vi "Get Settings.vi"(10 "VI path":path, 11 "switches":cluster{"switch":string, "argument":string}[](array[cluster])) -> (3 "settings":T1)   [LabVIEW 2017]
doc: "Prepares information necessary to create a new icon."
uses:
  CTLs/Settings.ctl
  CTLs/Template Frame.ctl
  CTLs/Text Format.ctl
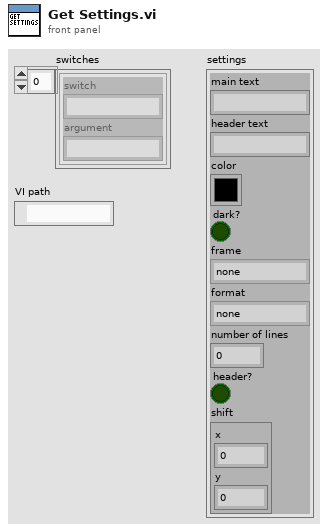
[diagram p1: front panel]
types:
  T1 = typedef "Settings.ctl" = cluster{"main text":string, "header text":string, "color":u32, "dark?":bool, "frame":T2, "format":T3, "number of lines":i32, "header?":bool, "shift":cluster{"x":i16, "y":i16}}
  T2 = typedef "Template Frame.ctl" = enum16{"none", "compact lib"}
  T3 = typedef "Text Format.ctl" = enum16{"none"}
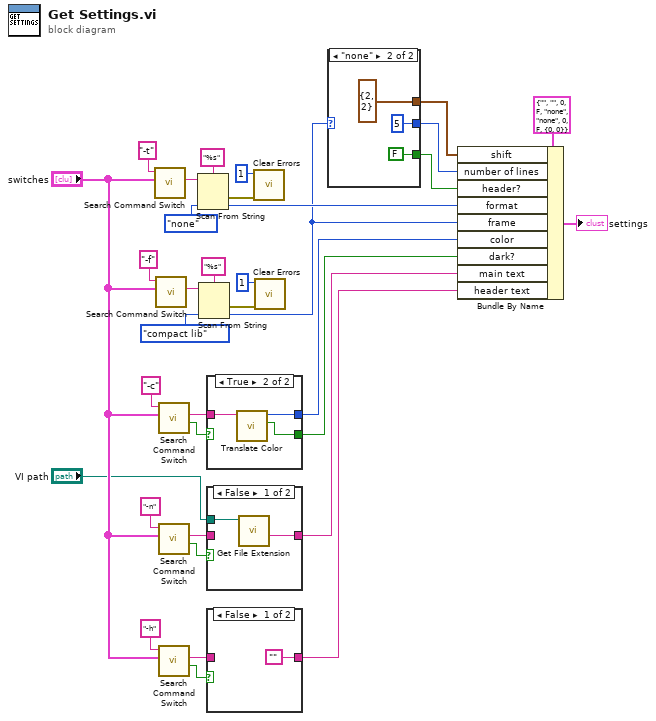
[diagram p0: block diagram]
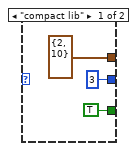
[diagram p2: hidden frame]
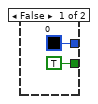
[diagram p5: hidden frame]
diagram:
  n1 = call "Search Command Switch.vi"("switches"="switches", "switch in"="-t") -> ("argument"=w22:string)  [unwired: 7 in, 2 out]
  n2 = call "Search Command Switch.vi"("switches"="switches", "switch in"="-f") -> ("argument"=w33:string)  [unwired: 7 in, 2 out]
  n3 = call "Search Command Switch.vi"("switches"="switches", "switch in"="-c") -> ("found?"=w26:bool, "argument"=w27:string)  [unwired: 7 in, 1 out]
  n4 = call "Search Command Switch.vi"("switches"="switches", "switch in"="-n") -> ("found?"=w19:bool, "argument"=w18:string)  [unwired: 7 in, 1 out]
  n5 = call "Search Command Switch.vi"("switches"="switches", "switch in"="-h") -> ("found?"=w14:bool, "argument"=w15:string)  [unwired: 7 in, 1 out]
  n6 = Scan From String(format string="%s", input string=w22, default 1=Text_Format."none" ("format")) -> (error out=w24:errorcluster, output 1=w11:T3)  [unwired: 2 in, 2 out]
  n7 = Scan From String(format string="%s", input string=w33, default 1=Template_Frame."compact lib" ("frame")) -> (error out=w30:errorcluster, output 1=w4:T2)  [unwired: 2 in, 2 out]
  n8 = case shown="True" w26 {
    tunnel: w27 -> [_ w39]
    tunnel: [u32 0 w38] -> w7
    tunnel: [TRUE ("dark?") w37] -> w8
    frame False {
    }
    frame True {
      n9 = call "Translate Color.vi"("color string"=w39) -> ("dark?"=w37:bool, "color"=w38:u32)  [unwired: 9 in]
    }
  }
  n10 = case shown="False" w19 {
    tunnel: w18 -> [_ w42]
    tunnel: [w41 w42] -> w9
    tunnel: "VI path" -> [w40 _]
    frame False {
      n11 = call <vilib>:"Get File Extension.vi"("file"=w40) -> ("filename without extension"=w41:string)  [unwired: 6 in, 4 out]
    }
    frame True {
    }
  }
  n12 = case shown="False" w14 {
    tunnel: w15 -> [_ w44]
    tunnel: ["" w44] -> w10
    frame False {
    }
    frame True {
    }
  }
  n13 = call <vilib>:"Clear Errors.vi"("error in (no error)"=w24, "specific error code to clear (0: all)"=1) -> ()  [unwired: 4 in, 2 out]
  n14 = call <vilib>:"Clear Errors.vi"("error in (no error)"=w30, "specific error code to clear (0: all)"=1) -> ()  [unwired: 4 in, 2 out]
  n15 = case shown="\"none\"" w4 {
    tunnel: [3 ("number of lines") 5 ("number of lines")] -> w3
    tunnel: [TRUE FALSE] -> w2
    tunnel: [cluster{"x":i16, "y":i16} {"x"=2, "y"=10} ("shift") cluster{"x":i16, "y":i16} {"x"=2, "y"=2} ("shift")] -> w1
    frame "compact lib" {
    }
    frame "none" {
    }
  }
  n16 = Bundle By Name(cluster=T1 {"main text"="", "header text"="", "color"=0, "dark?"=FALSE, "frame"=enum."none", "format"=enum."none", "number of lines"=0, "header?"=FALSE, "shift"={"x"=0, "y"=0}}, "shift"=w1, "number of lines"=w3, "header?"=w2, "format"=w11, "frame"=w4, "color"=w7, "dark?"=w8, "main text"=w9, "header text"=w10) -> (→"settings":T1)
